vi "readManual.vi"(6 "readingRate(ms)":u32=100, 8 "error in (no error)":errorcluster, 9 "Reading Option (0: Latest)":i32, 10 "Electrometer in":refnum<class "Electrometer.lvclass">, 11 "ReadyState in":refnum<class "ReadyState.lvclass">) -> (0 "error out":errorcluster, 1 "Electrometer out":refnum<class "Electrometer.lvclass">, 2 "result":dbl[](array[numeric]), 3 "ReadyState out":refnum<class "ReadyState.lvclass">)   [LabVIEW 2016, in "ReadyState.lvclass"]
uses:
  ReadyState.lvclass
  Electrometer.lvclass
panel:
  out "local stop":bool
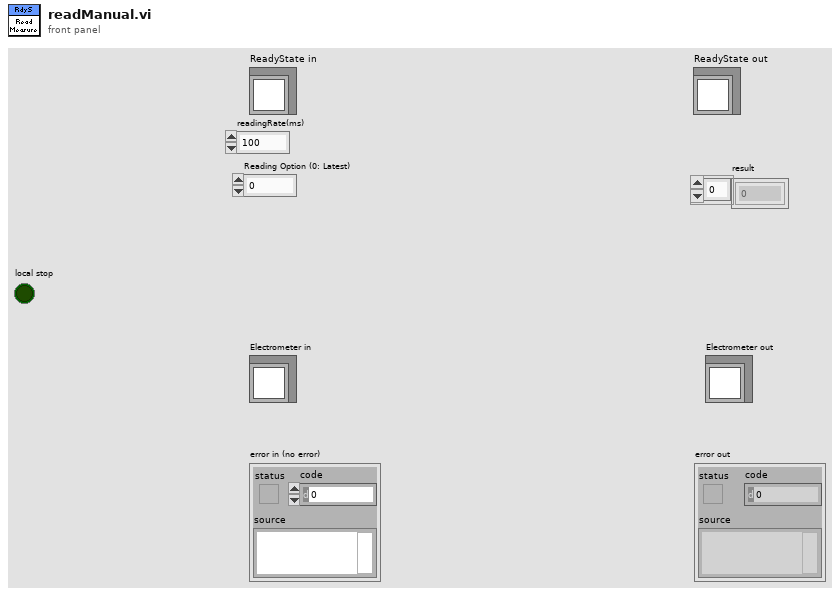
[diagram p1: front panel]
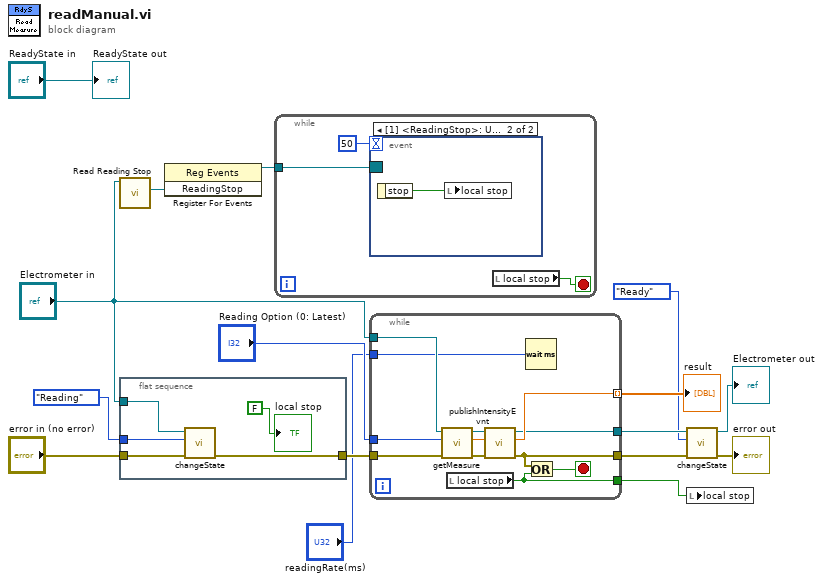
[diagram p0: block diagram]
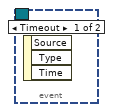
[diagram p2: hidden frame]
diagram:
  n1 = call-dynamic "Read Reading Stop.vi"("Electrometer in"="Electrometer in") -> ("ReadingStop"=w13:refnum<user-event>)  [unwired: 8 in, 2 out]
  n2 = flat-sequence {
    tunnel: "error in (no error)" -> [w19]
    tunnel: [w20] -> w11
    tunnel: "Electrometer in" -> [w18]
    tunnel: enum16{"Configuring", "Ready", "Reading"}."Reading" ("newState") -> [w17]
    frame #0 {
      n3 = call-dynamic "changeState.vi"("error in (no error)"=w19, "State"=w17, "Electrometer in"=w18) -> ("error out"=w20:errorcluster)  [unwired: 7 in, 1 out]
      "local stop" <- FALSE ("local stop")
    }
  }
  n4 = register-events(w13) -> (reference out=w12:refnum<event-registration>)  [unwired: 2 in, 1 out]
  n5 = while {
    tunnel: w12 -> [w23]
    stop <- w24 stop-if-true
    n6 = event shown="[1] <ReadingStop>: User Event" {
      selector: w23 -> [_ _]
      dyn-events: _ -> [_ _]
      timeout: 50 -> [_ _]
      event Timeout {
        n7 = event-data() -> ()  [unwired: 1 in, 3 out]
      }
      event User Event {
        n8 = event-data() -> ("stop"=w25:bool)  [unwired: 1 in]
        n9 = local write "local stop"(w25) -> ()
      }
    }
    n10 = local read "local stop"() -> (w24:bool)
  }
  n11 = while {
    tunnel: "Electrometer in" -> [w37]
    tunnel: w11 -> [w36]
    tunnel: [w28] -> w4
    tunnel: [w32] -> w5
    tunnel: "Reading Option (0: Latest)" -> [w34]
    tunnel: [w31] -> w14 mode=indexing
    tunnel: [w27] -> w9
    tunnel: "readingRate(ms)" -> [w26]
    stop <- w35 stop-if-true
    n12 = call "getMeasure.vi"("error in (no error)"=w36, "Reading Option (0: Latest)"=w34, "Electrometer in"=w37) -> ("error out"=w33:errorcluster, "Measure"=w30:dbl, "Electrometer out"=w29:refnum<class "Electrometer.lvclass">)  [unwired: 6 in]
    n13 = local read "local stop"() -> (w27:bool)
    n14 = call-dynamic "publishIntensityEvnt.vi"("error in (no error)"=w33, "Intensity"=w30, "Electrometer in"=w29) -> ("error out"=w32:errorcluster, "Intensity out"=w31:dbl, "Electrometer out"=w28:refnum<class "Electrometer.lvclass">)  [unwired: 6 in]
    n15 = Wait (ms)(milliseconds to wait=w26) -> ()  [unwired: 1 out]
    n16 = Or(x=w32, y=w27) -> (x .or. y?=w35:bool)
  }
  "result" <- w14
  n17 = call-dynamic "changeState.vi"("error in (no error)"=w5, "State"=enum16{"Configuring", "Ready", "Reading"}."Ready" ("newState"), "Electrometer in"=w4) -> ("error out"=→"error out":errorcluster, "Electrometer out"=→"Electrometer out":refnum<class "Electrometer.lvclass">)  [unwired: 7 in]
  n18 = local write "local stop"(w9) -> ()
  "ReadyState out" <- "ReadyState in"
